vi "Hardware Scan.vi"(8 "error in (no error)":errorcluster, 11 "Controller in":refnum<class "Controller.lvclass">) -> (0 "error out":errorcluster, 3 "Controller out":refnum<class "Controller.lvclass">)   [LabVIEW 2016, in "Controller Actor.lvlib" / "Controller.lvclass"]
uses:
  <userlib>/Common Components/Controller/Controller.lvclass
  C:/Program Files (x86)/National Instruments/LabVIEW 2016/vi.lib/ActorFramework/Actor/Actor.lvclass
  <userlib>/Common Components/Hardware/Abstract Hardware/Hardware.lvclass
  <userlib>/Common Components/Controller UI/Update DT event data.ctl
  <userlib>/Common Components/Controller UI/Update DT Cmd.ctl
  <userlib>/Common Components/Controller/Controller.lvclass/Controller.ctl
  <vilib>/ActorFramework/Actor/Actor.lvclass/Actor.ctl
  <vilib>/ActorFramework/Message Enqueuer/Message Enqueuer.lvclass/Message Enqueuer.ctl
  <userlib>/Common Components/Controller UI Messages/Update DT Event Msg/Update DT Event Msg.lvclass/Update DT Event Msg.ctl
  <userlib>/Common Components/Controller/Accessors/Read Root Path.vi
  <vilib>/ActorFramework/Message Enqueuer/Init from Existing Queue.vi
  <vilib>/ActorFramework/Message Enqueuer/Enqueue.vi
  <userlib>/Common Components/Controller UI Messages/Update DT Event Msg/Update DT Event Msg.lvclass
  C:/Program Files (x86)/National Instruments/LabVIEW 2016/vi.lib/ActorFramework/Message/Message.lvclass
  <vilib>/ActorFramework/Message Priority Queue/Priority Enqueue.vi
  <vilib>/ActorFramework/Message Enqueuer/Message Enqueuer.lvclass
  <vilib>/ActorFramework/Actor/Actor.lvclass
  <userlib>/Common Components/Controller/Messages/Log Status/Log Status.lvclass
  <userlib>/Common Components/Controller UI/Controller UI.lvclass
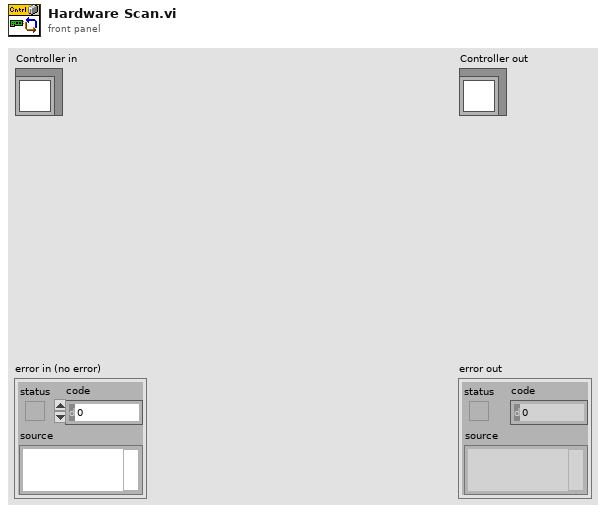
[diagram p1: front panel]
types:
  T1 = typedef "Controller UI.lvlib/Controller UI.lvclass/Update DT event data.ctl" = cluster{"Cmd":T2, "Data Array":variant[]}
  T2 = typedef "Controller UI.lvlib/Controller UI.lvclass/Update DT Cmd.ctl" = enum16{"Update HWtype\\HWplugin array", "Update Checked-out", "Update COMM Status", "Load DevInfo from File", "Save DevInfo to File", "Update COMM Address List"}
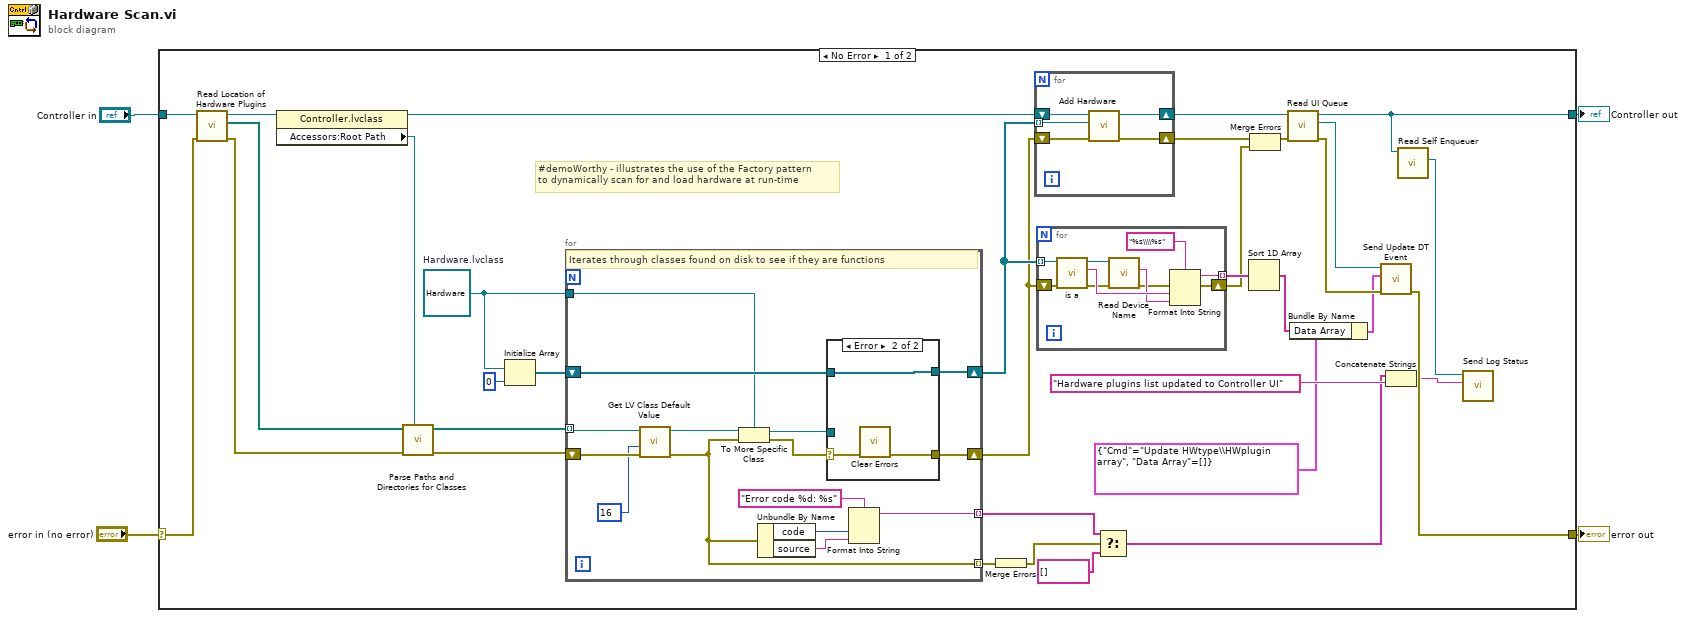
[diagram p0: block diagram]
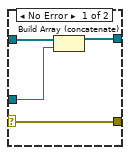
[diagram p2: hidden frame]
diagram:
  n1 = case shown="No Error" "error in (no error)" {
    selector: "error in (no error)" -> [w34 w77]
    tunnel: [w19 w77] -> w3
    tunnel: [w16 w76] -> w1
    tunnel: "Controller in" -> [w38 w76]
    frame No Error {
      w37 = refnum<class "Hardware.lvclass"> refnum  # Hardware.lvclass
      # "#demoWorthy - illustrates the use of the Factory pattern\nto dynamically scan for and load hardware at run-time"
      n2 = call <userlib>:"Read Location of Hardware Plugins.vi"("error in (no error)"=w34, "Controller in"=w38) -> ("error out"=w31:errorcluster, "Array of Hardware Paths"=w32:path[], "Controller out"=w28:refnum<class "Controller.lvclass">)  [unwired: 7 in]
      n3 = property class="Controller.lvclass"(reference=w28) -> (reference out=w26:refnum<class "Controller.lvclass">, "Accessors:Root Path"=w27:path)  [unwired: 1 in, 1 out]
      n4 = call <userlib>:"Parse Paths and Directories for Classes.vi"("base path"=w27, "error in (no error)"=w31, "Array of paths (folders to scan or explicit files)"=w32) -> ("error out"=w30:errorcluster, "All Files in Dir"=w29:path[])  [unwired: 7 in]
      n5 = Initialize Array(w37, 0 ("dimension size")) -> (w36:refnum<class "Hardware.lvclass">[])
      n6 = for {
        tunnel: w29 -> [w63] mode=indexing
        shift-right: [w67] -> w25
        shift-left: w36 -> [w65]
        shift-right: [w64] -> w24
        shift-left: w30 -> [w66]
        tunnel: w37 -> [w61]
        tunnel: [w55] -> w7 mode=indexing
        tunnel: [w54] -> w9 mode=indexing
        # "Iterates through classes found on disk to see if they are functions"
        n7 = call <vilib>:"Get LV Class Default Value.vi"("error in (no error)"=w66, "options"=u32 16, "class path"=w63) -> ("error out"=w54:errorcluster, "object"=w62:refnum<class>)  [unwired: 7 in]
        n8 = To More Specific Class(target class=w61, reference=w62, error in=w54) -> (specific class reference=w68:refnum<class "Hardware.lvclass">, error out=w60:errorcluster)
        n9 = Unbundle By Name(w54) -> ("code"=w57:i32, "source"=w56:string)
        n10 = case shown="Error" w60 {
          selector: w60 -> [w69 w74]
          tunnel: w68 -> [w70 _]
          tunnel: [w72 w75] -> w67
          tunnel: w65 -> [w71 w75]
          tunnel: [w69 w73] -> w64
          frame No Error {
            n11 = Build Array (concatenate)(w71, w70) -> (w72:refnum<class "Hardware.lvclass">[])
          }
          frame Error {
            n12 = call <vilib>:"Clear Errors.vi"("error in (no error)"=w74) -> ("error out"=w73:errorcluster)  [unwired: 5 in, 1 out]
          }
        }
        n13 = Format Into String(format string="Error code %d: %s", w57, w56) -> (resulting string=w55:string)  [unwired: 2 in, 1 out]
      }
      n14 = Merge Errors(w9) -> (w8:errorcluster)
      n15 = for {
        shift-right: [w52] -> w22
        shift-left: w26 -> [w53]
        tunnel: w25 -> [w51] mode=indexing
        shift-right: [w49] -> w33
        shift-left: w24 -> [w50]
        n16 = call <userlib>:"Add Hardware.vi"("error in (no error)"=w50, "Hardware.lvclass"=w51, "Controller in"=w53) -> ("error out"=w49:errorcluster, "Controller out"=w52:refnum<class "Controller.lvclass">)  [unwired: 7 in]
      }
      n17 = for {
        tunnel: w25 -> [w48] mode=indexing
        shift-right: [w40] -> w17
        shift-left: w24 -> [w43]
        tunnel: [w39] -> w23 mode=indexing
        n18 = call-dynamic "is a.vi"("error in (no error)"=w43, "Hardware in"=w48) -> ("error out"=w42:errorcluster, "is a"=w45:string, "Hardware out"=w47:refnum<class "Hardware.lvclass">)  [unwired: 7 in]
        n19 = call <userlib>:"Read Device Name.vi"("error in (no error)"=w42, "Analog in"=w47) -> ("error out"=w41:errorcluster, "Device Name"=w44:string)  [unwired: 7 in, 1 out]
        n20 = Format Into String(format string="%s\\\\%s", error in=w41, w45, w44) -> (resulting string=w39:string, error out=w40:errorcluster)  [unwired: 1 in]
      }
      n21 = Select(t=w7, s=w8, f=string[] []) -> (s? t:f=w5:string[])
      n22 = Sort 1D Array(array=w23) -> (sorted array=w11:string[])
      n23 = Merge Errors(w33, w17) -> (w18:errorcluster)
      n24 = call <userlib>:"Read UI Queue.vi"("error in (no error)"=w18, "UI Controller in"=w22) -> ("error out"=w20:errorcluster, "UI Queue"=w21:refnum<class "Message Enqueuer.lvclass">, "UI Controller out"=w16:refnum<class "Controller.lvclass">)  [unwired: 7 in]
      n25 = Bundle By Name(cluster=T1 {"Cmd"=enum."Update HWtype\\HWplugin array", "Data Array"=[]} ("event data"), "Data Array"=w11) -> (w12:T1)
      n26 = call <userlib>:"Send Update DT Event.vi"("error in (no error)"=w20, "event data"=w12, "Message Enqueuer"=w21) -> ("error out"=w19:errorcluster)  [unwired: 7 in, 1 out]
      n27 = Concatenate Strings(w5, "Hardware plugins list updated to Controller UI" ("String")) -> (w10:string)
      n28 = call <vilib>:"Read Self Enqueuer.vi"("Actor"=w16) -> ("Self Enqueuer"=w15:refnum<class "Message Enqueuer.lvclass">)  [unwired: 10 in]
      n29 = call <userlib>:"Send Log Status.vi"("String"=w10, "Message Enqueuer in"=w15) -> ()  [unwired: 8 in, 2 out]
    }
    frame Error {
    }
  }
  "error out" <- w3
  "Controller out" <- w1
